vi "ClusterToJSON.vi"() -> ()   [LabVIEW 2022 SP3, in "Test_Flux_Capacitor.lvlib" / "Test_Flux_Capacitor.lvclass"]
uses:
  Test_Flux_Capacitor.lvclass
  ParameterTypes/485_Loopback.ctl
  ParameterTypes/MeasureVoltage.ctl
  ParameterTypes/DMM_DCV.vi
panel:
  in  "Parameter_Type 2":T1={"Switch"="", "Wait (msec)"=0, "Scale"=0.0, "DMM_DCV"={"Range "=enum."Auto", "Resolution"=enum."Default", "Samples"=1, "dt (s)"=0.0, "Timeout (s)"=10000.0}}
  in  "Meas_Speed":enum16{"Slow", "Fast"}(ring)=enum."Fast"
  out "JSON String":string
  in  "Parameter_Type":T3
  # "`"
  # "{\n    \"Pre_Switch\":\"con_c108_c109\",\n    \"Post_Switch\":\"dis_c108_c109\",\n    \"Wait (msec)\":2000,\n    \"LCR\":{\n        \"F_(Hz)\":35,\n        \"Range\":\"Auto\",\n        \"Signal_Level\":\"1Vrms\",\n        \"Function\":\"Cp-Q\",\n        \"Meas_Speed\":\"Slow\"\n    },\n    \"Scale\":1000000\n}"
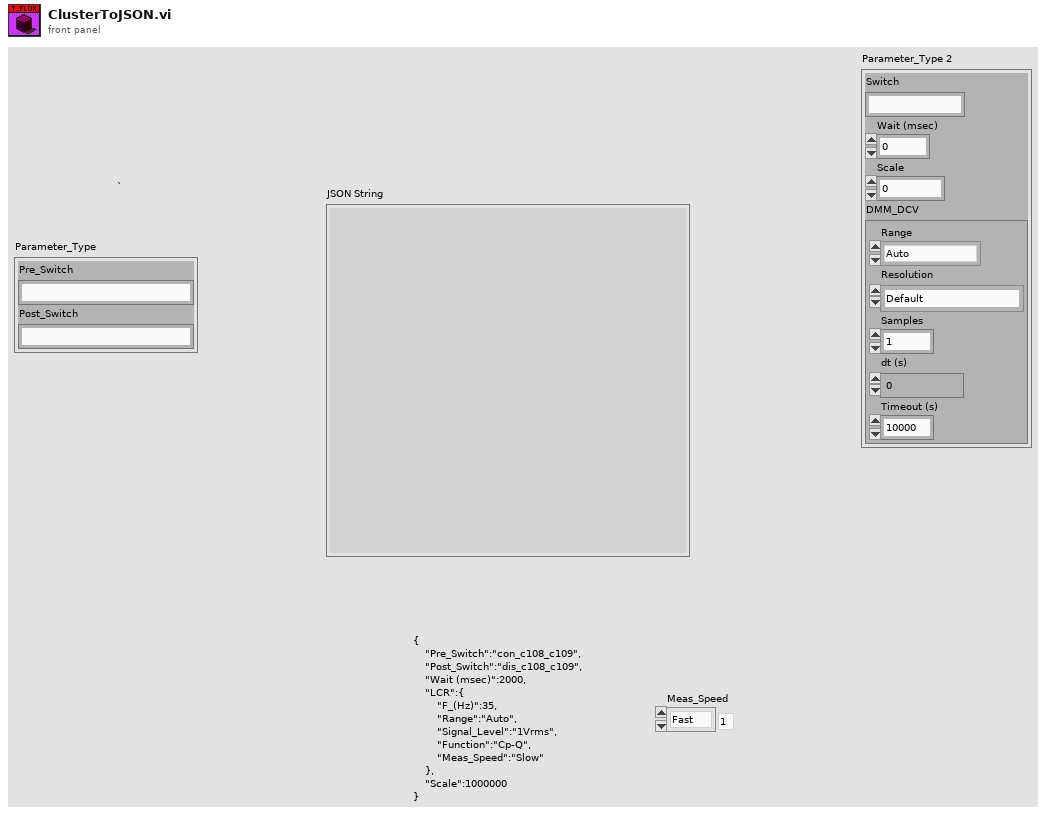
[diagram p1: front panel]
types:
  T1 = typedef "Test_Flux_Capacitor.lvlib/Test_Flux_Capacitor.lvclass/MeasureVoltage.ctl" = cluster{"Switch":string, "Wait (msec)":u32, "Scale":dbl, "DMM_DCV":T2}
  T2 = typedef "Test_Flux_Capacitor.lvlib/Test_Flux_Capacitor.lvclass/DMM_DCV.vi" = cluster{"Range ":enum16{"100 mV", "1 V", "10 V", "100 V", "300 V", "Auto", "Minimum", "Maximum"}, "Resolution":enum16{"4 1/2", "5 1/2", "6 1/2", "Least", "Highest", "Default"}, "Samples":u32, "dt (s)":dbl, "Timeout (s)":dbl}
  T3 = typedef "Test_Flux_Capacitor.lvlib/Test_Flux_Capacitor.lvclass/485_Loopback.ctl" = cluster{"Pre_Switch":string, "Post_Switch":string}
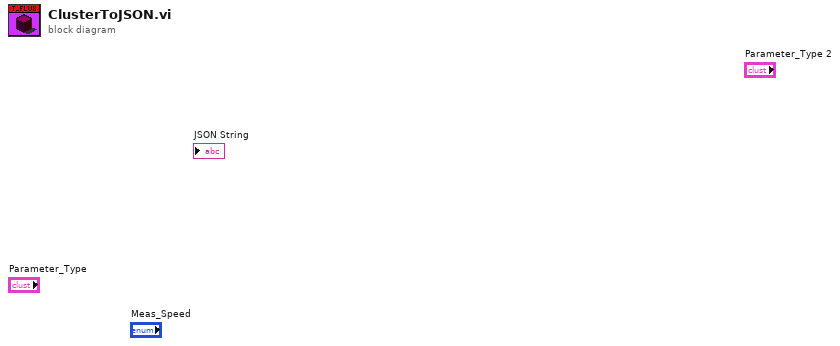
[diagram p0: block diagram]
diagram:
